vi "Untitled 1.vi"() -> ()   [LabVIEW 2019]
panel:
  in  "stop":bool
  in  "Activate":bool
  out "R_4":bool
  out "Y_4":bool
  out "G_4":bool
  out "R_3":bool
  out "Y_3":bool
  out "G_3":bool
  out "R_2":bool
  out "Y_2":bool
  out "G_2":bool
  out "R_1":bool
  out "Y_1":bool
  out "G_1":bool
  # "Labview Traffic Light"
  # "Siwar Gharbi"
  # "Voie 3"
  # "Voie 1"
  # "Voie 2"
  # "Voie 4"
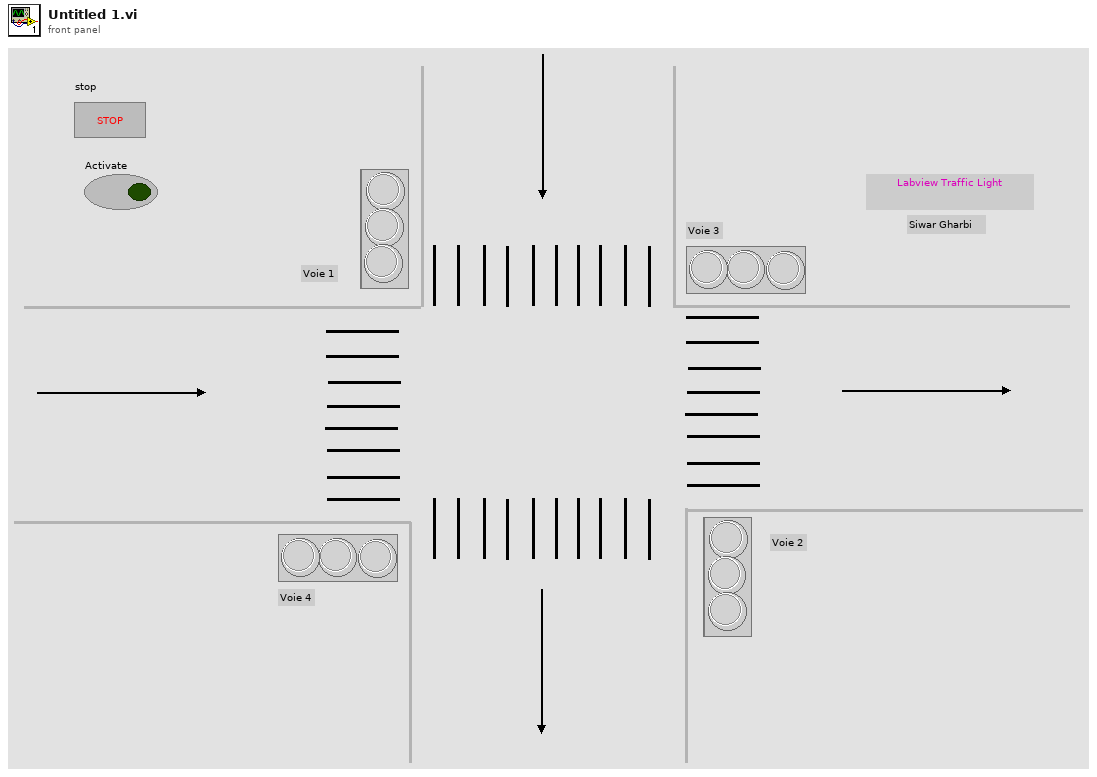
[diagram p1: front panel]
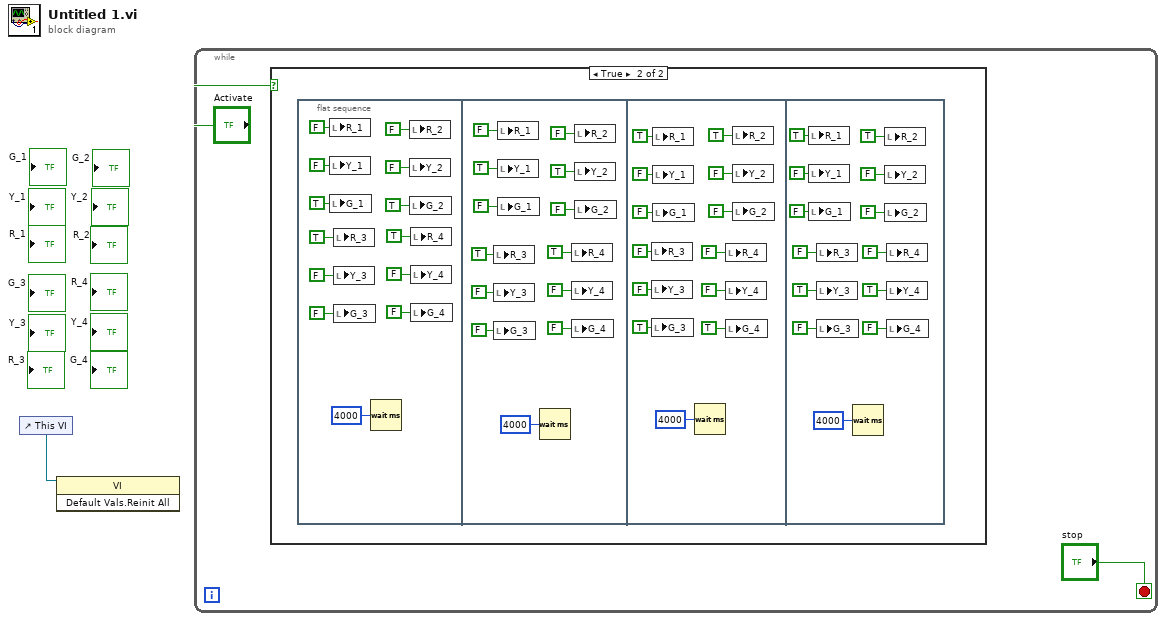
[diagram p0: block diagram]
diagram:
  n1 = control-ref of="This VI"() -> (w1:refnum<vi>)
  n2 = invoke class="VI" method="Default Vals.Reinit All"(reference=w1) -> ()  [unwired: 2 in, 3 out]
  n3 = while {
    stop <- "stop" stop-if-true
    n4 = case shown="True" "Activate" {
      frame False {
      }
      frame True {
        n5 = flat-sequence {
          frame #0 {
            n6 = local write "R_1"(FALSE ("R_1")) -> ()
            n7 = local write "Y_1"(FALSE ("Y_1")) -> ()
            n8 = local write "G_1"(TRUE ("G_1")) -> ()
            n9 = local write "R_3"(TRUE ("R_3")) -> ()
            n10 = local write "Y_3"(FALSE ("Y_3")) -> ()
            n11 = local write "G_3"(FALSE ("G_3")) -> ()
            n12 = Wait (ms)(milliseconds to wait=u32 4000) -> ()  [unwired: 1 out]
            n13 = local write "R_2"(FALSE ("R_2")) -> ()
            n14 = local write "Y_2"(FALSE ("Y_2")) -> ()
            n15 = local write "G_2"(TRUE ("G_2")) -> ()
            n16 = local write "R_4"(TRUE ("R_4")) -> ()
            n17 = local write "Y_4"(FALSE ("Y_4")) -> ()
            n18 = local write "G_4"(FALSE ("G_4")) -> ()
          }
          frame #1 {
            n19 = local write "R_3"(TRUE ("R_3")) -> ()
            n20 = local write "Y_3"(FALSE ("Y_3")) -> ()
            n21 = local write "G_3"(FALSE ("G_3")) -> ()
            n22 = local write "R_1"(FALSE ("R_1")) -> ()
            n23 = local write "Y_1"(TRUE ("Y_1")) -> ()
            n24 = local write "G_1"(FALSE ("G_1")) -> ()
            n25 = Wait (ms)(milliseconds to wait=u32 4000) -> ()  [unwired: 1 out]
            n26 = local write "R_4"(TRUE ("R_4")) -> ()
            n27 = local write "Y_4"(FALSE ("Y_4")) -> ()
            n28 = local write "G_4"(FALSE ("G_4")) -> ()
            n29 = local write "R_2"(FALSE ("R_2")) -> ()
            n30 = local write "Y_2"(TRUE ("Y_2")) -> ()
            n31 = local write "G_2"(FALSE ("G_2")) -> ()
          }
          frame #2 {
            n32 = local write "R_3"(FALSE ("R_3")) -> ()
            n33 = local write "Y_3"(FALSE ("Y_3")) -> ()
            n34 = local write "G_3"(TRUE ("G_3")) -> ()
            n35 = local write "R_1"(TRUE ("R_1")) -> ()
            n36 = local write "Y_1"(FALSE ("Y_1")) -> ()
            n37 = local write "G_1"(FALSE ("G_1")) -> ()
            n38 = Wait (ms)(milliseconds to wait=u32 4000) -> ()  [unwired: 1 out]
            n39 = local write "R_4"(FALSE ("R_4")) -> ()
            n40 = local write "Y_4"(FALSE ("Y_4")) -> ()
            n41 = local write "G_4"(TRUE ("G_4")) -> ()
            n42 = local write "R_2"(TRUE ("R_2")) -> ()
            n43 = local write "Y_2"(FALSE ("Y_2")) -> ()
            n44 = local write "G_2"(FALSE ("G_2")) -> ()
          }
          frame #3 {
            n45 = local write "R_1"(TRUE ("R_1")) -> ()
            n46 = local write "Y_1"(FALSE ("Y_1")) -> ()
            n47 = local write "G_1"(FALSE ("G_1")) -> ()
            n48 = local write "R_3"(FALSE ("R_3")) -> ()
            n49 = local write "Y_3"(TRUE ("Y_3")) -> ()
            n50 = local write "G_3"(FALSE ("G_3")) -> ()
            n51 = Wait (ms)(milliseconds to wait=u32 4000) -> ()  [unwired: 1 out]
            n52 = local write "R_2"(TRUE ("R_2")) -> ()
            n53 = local write "Y_2"(FALSE ("Y_2")) -> ()
            n54 = local write "G_2"(FALSE ("G_2")) -> ()
            n55 = local write "R_4"(FALSE ("R_4")) -> ()
            n56 = local write "Y_4"(TRUE ("Y_4")) -> ()
            n57 = local write "G_4"(FALSE ("G_4")) -> ()
          }
        }
      }
    }
  }
